vi "changeCursorPosition.vi"(4 "Cursor Y position":dbl, 5 "Cursor X position":dbl, 6 "Cursos id":i32, 7 "Intensity Graph 2":refnum<vi>) -> (2 "error out":errorcluster, 3 "reference out":refnum<vi>)   [LabVIEW 2014]
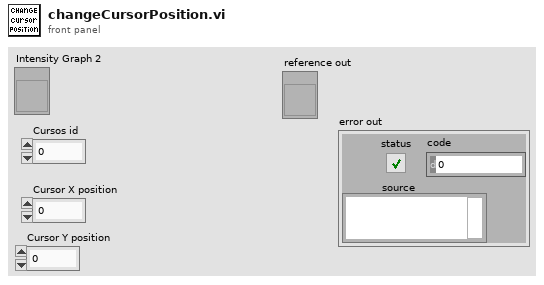
[diagram p1: front panel]
types:
  T1 = typedef "LVCursorListTypeDef.ctl" = cluster{"Name":string, "Color":u32, "Style":u8, "Point Style":u8, "Name Visible":bool, "Allow Drag":bool, "Cursor Mode":u32, "Plot":i32, "Index":i32, "Position":cluster{"X":dbl, "Y":dbl}, "X Scale":u32, "Y Scale":u32, "Watch Plots":i32[], "Watch All Plots":bool, "Plot Area":i32, "Label Offset":cluster{"X":dbl, "Y":dbl}}[]
  T2 = cluster{"Name":string, "Color":u32, "Style":u8, "Point Style":u8, "Name Visible":bool, "Allow Drag":bool, "Cursor Mode":u32, "Plot":i32, "Index":i32, "Position":cluster{"X":dbl, "Y":dbl}, "X Scale":u32, "Y Scale":u32, "Watch Plots":i32[], "Watch All Plots":bool, "Plot Area":i32, "Label Offset":cluster{"X":dbl, "Y":dbl}}
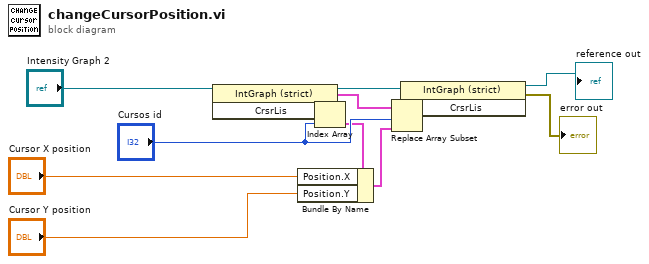
[diagram p0: block diagram]
diagram:
  n1 = property on="Property Node" class="IntGraph (strict)"(reference="Intensity Graph 2") -> (reference out=w11:refnum<vi>, "CrsrLis"=w5:T1)  [unwired: 1 in, 1 out]
  n2 = Index Array(array=w5, index="Cursos id") -> (element=w4:T2)
  n3 = Bundle By Name(cluster=w4, "Position.X"="Cursor X position", "Position.Y"="Cursor Y position") -> (w8:T2)
  n4 = Replace Array Subset(array=w5, new element=w8, index="Cursos id") -> (w6:T1)
  n5 = property on="Property Node" class="IntGraph (strict)"(reference=w11, "CrsrLis"=w6) -> (reference out=→"reference out":refnum<vi>, error out=→"error out":errorcluster)  [unwired: 1 in]
